vi "Pre Launch Init.vi"(11 "Display Console in":refnum<class "Sensor Interface.lvclass">) -> (0 "error out":errorcluster, 3 "Display Console out":refnum<class "Sensor Interface.lvclass">)   [LabVIEW 2019, in "Sensor Interface Actor.lvlib" / "Sensor Interface.lvclass"]
doc: "(<B>Filename</B>: Actor Framework.lvlib:Actor.lvclass:Pre Launch Init.vi)\n\nDefines behavior that occurs after the Launch Nested Actor method is invoked but before the actor's Actor Core method begins running.\n\nBy default, this method does nothing. A descendant class may override it to define behavior."
uses:
  Sensor Interface.lvclass
  Sensor Interface.lvclass/Sensor Interface.ctl
  Abstract Sensor Interface Actor/Abstract Sensor Interface/Abstract Sensor Interface.lvclass
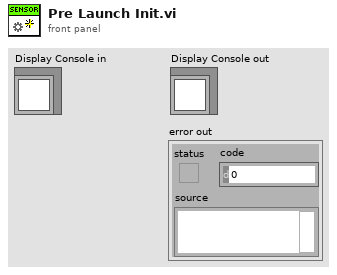
[diagram p1: front panel]
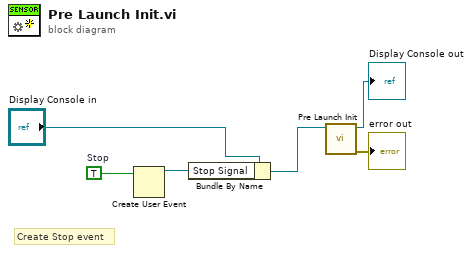
[diagram p0: block diagram]
diagram:
  w4 = TRUE  # Stop
  # "Create Stop event"
  n1 = Create User Event(user event datatype=w4) -> (user event=w3:refnum<user-event>)  [unwired: 1 in, 1 out]
  n2 = Bundle By Name(cluster="Display Console in", "Stop Signal"=w3) -> (w1:refnum<class "Sensor Interface.lvclass">)
  n3 = call-parent "Pre Launch Init.vi"("Actor in"=w1) -> ("error out"=→"error out":errorcluster, "Actor out"=→"Display Console out":refnum<class "Sensor Interface.lvclass">)  [unwired: 9 in]
